vi "Convertir_WResponse8bits_of_string_ToBool.vi"(11 "Response 8bit":string) -> (3 "appended array":bool[](array[boolean]))   [LabVIEW 2019]
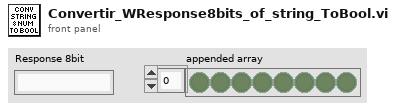
[diagram p1: front panel]
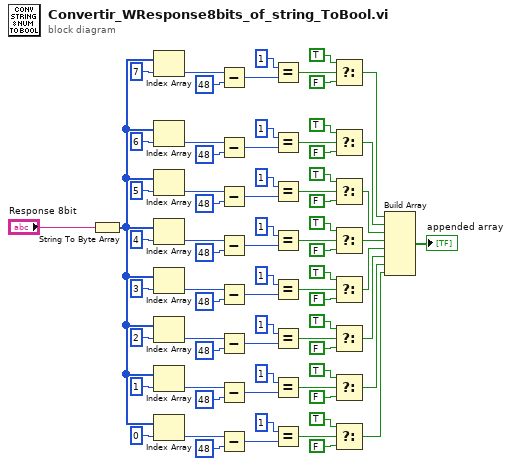
[diagram p0: block diagram]
diagram:
  n1 = String To Byte Array(string="Response 8bit") -> (unsigned byte array=w10:u8[])
  n2 = Index Array(array=w10, index=7) -> (element=w35:u8)
  n3 = Index Array(array=w10, index=6) -> (element=w33:u8)
  n4 = Index Array(array=w10, index=5) -> (element=w31:u8)
  n5 = Index Array(array=w10, index=4) -> (element=w29:u8)
  n6 = Index Array(array=w10, index=3) -> (element=w27:u8)
  n7 = Index Array(array=w10, index=2) -> (element=w25:u8)
  n8 = Index Array(array=w10, index=1) -> (element=w23:u8)
  n9 = Index Array(array=w10, index=0) -> (element=w20:u8)
  n10 = Subtract(x=w35, y=u8 48) -> (x-y=w70:u8)
  n11 = Subtract(x=w33, y=u8 48) -> (x-y=w65:u8)
  n12 = Subtract(x=w31, y=u8 48) -> (x-y=w60:u8)
  n13 = Subtract(x=w29, y=u8 48) -> (x-y=w55:u8)
  n14 = Subtract(x=w27, y=u8 48) -> (x-y=w50:u8)
  n15 = Subtract(x=w25, y=u8 48) -> (x-y=w45:u8)
  n16 = Subtract(x=w23, y=u8 48) -> (x-y=w36:u8)
  n17 = Subtract(x=w20, y=u8 48) -> (x-y=w75:u8)
  n18 = Equal?(x=u8 1, y=w70) -> (x = y?=w67:bool)
  n19 = Equal?(x=u8 1, y=w65) -> (x = y?=w62:bool)
  n20 = Equal?(x=u8 1, y=w60) -> (x = y?=w57:bool)
  n21 = Equal?(x=u8 1, y=w55) -> (x = y?=w52:bool)
  n22 = Equal?(x=u8 1, y=w50) -> (x = y?=w47:bool)
  n23 = Equal?(x=u8 1, y=w45) -> (x = y?=w42:bool)
  n24 = Equal?(x=u8 1, y=w36) -> (x = y?=w38:bool)
  n25 = Equal?(x=u8 1, y=w75) -> (x = y?=w72:bool)
  n26 = Select(t=TRUE, s=w67, f=FALSE) -> (s? t:f=w2:bool)
  n27 = Select(t=TRUE, s=w62, f=FALSE) -> (s? t:f=w3:bool)
  n28 = Select(t=TRUE, s=w57, f=FALSE) -> (s? t:f=w4:bool)
  n29 = Select(t=TRUE, s=w52, f=FALSE) -> (s? t:f=w5:bool)
  n30 = Select(t=TRUE, s=w47, f=FALSE) -> (s? t:f=w6:bool)
  n31 = Select(t=TRUE, s=w42, f=FALSE) -> (s? t:f=w7:bool)
  n32 = Select(t=TRUE, s=w38, f=FALSE) -> (s? t:f=w8:bool)
  n33 = Select(t=TRUE, s=w72, f=FALSE) -> (s? t:f=w9:bool)
  n34 = Build Array(w2, w3, w4, w5, w6, w7, w8, w9) -> (→"appended array":bool[])
